vi "json2csv_no_invokes_of_dependencies.vi"() -> ()   [LabVIEW 2018]
uses:
  C:/Users/booko/Desktop/ENABLE/lv18_using_dll/dependencies/json2csv.dll
  dependencies/json2csv.dll
panel:
  out "jsonToCSV":string
  in  "jsonContent":string="[{\"x_Tx\":\"0,000\",\"y_Tx\":\"0,000\",\"z_Tx\":\"1,000\",\"th_Tx\":\"0,000\",\"phi_Tx\":\"0,000\",\"x_Rx\":\"0,000\",\"y_Rx\":\"0,000\",\"z_Rx\":\"1,000\",\"th_Rx\":\"0,000\",\"phi_Rx\":\"0,000\",\"f0\":\"2450000000,000\",\"BW\":\"20000000,000\",\"RX_custom_antenna\":\"\",\"TX_JX_custom_antenna\":\"\"}]"
  in  "error in (no error)":errorcluster
  out "error out":errorcluster={"status"=TRUE, "code"=1172, "source"="Invoke Node System.Reflection.TargetInvocationException: Obiekt docelowy wywołania zgłosił wyjątek.\n\tInner Exception: Newtonsoft.Json.JsonSerializationException: Unexpected JSON token when reading DataTable. Expected StartArray, got StartObject. Path '', line 1, position 1. <append><b>Newtonsoft.Json.JsonSerializationException</b> in json2csv_no_invokes_of_dependencies.vi"}
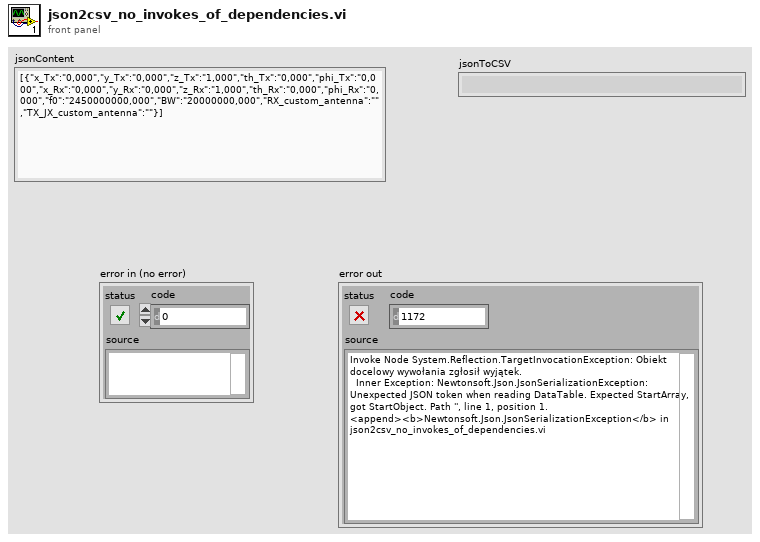
[diagram p1: front panel]
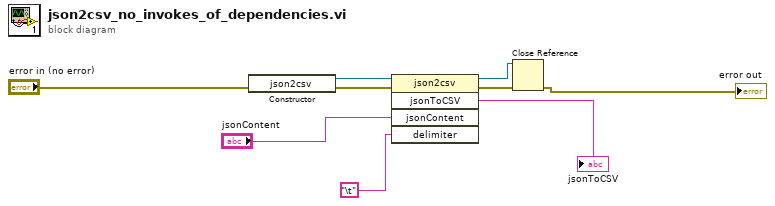
[diagram p0: block diagram]
diagram:
  n1 = constructor class="json2csv"(error in="error in (no error)") -> (reference out=w9:refnum<k24>, error out=w7:errorcluster)  [unwired: 2 in, 1 out]
  n2 = invoke class="json2csv" method="jsonToCSV"(reference=w9, error in=w7, "jsonContent"="jsonContent", "delimiter"="\t") -> (reference out=w8:refnum<k24>, error out=w6:errorcluster, "jsonToCSV"=→"jsonToCSV":string)  [unwired: 1 in, 2 out]
  n3 = Close Reference(reference=w8, error in (no error)=w6) -> (error out=→"error out":errorcluster)
